vi "判决.vi"(1 "判决门限":dbl, 2 "噪声数组":dbl[](array[numeric]), 3 "码元数组":dbl[](array[numeric])) -> (0 "错误计数":dbl)   [LabVIEW 2020]
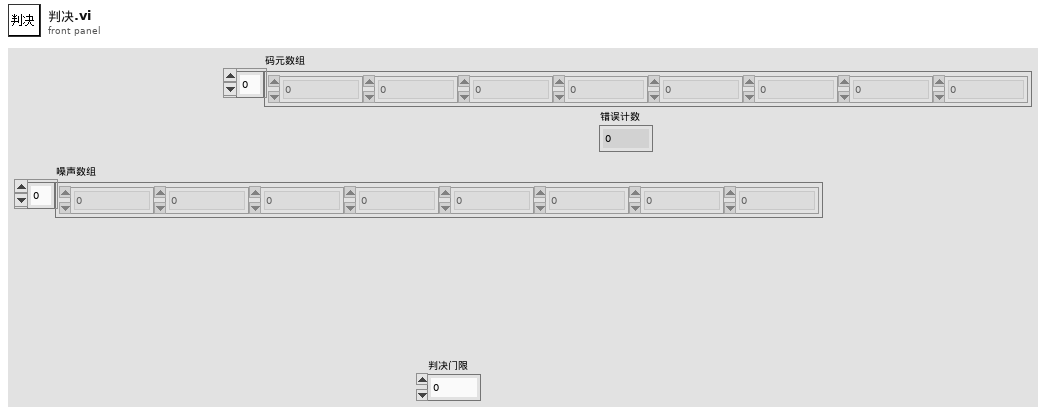
[diagram p1: front panel]
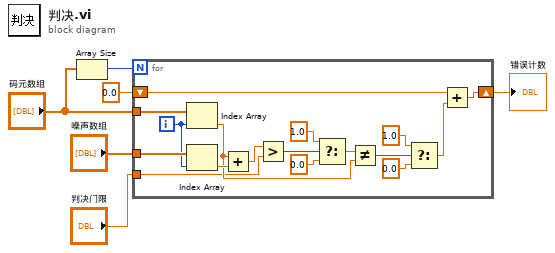
[diagram p0: block diagram]
diagram:
  n1 = Array Size(array="码元数组") -> (size(s)=w1:i32)
  n2 = for {
    N: w1 -> [_]
    tunnel: "噪声数组" -> [w19]
    shift-right: [w13] -> w3
    shift-left: 0.0 -> [w14]
    tunnel: "码元数组" -> [w8]
    tunnel: "判决门限" -> [w7]
    i -> [w10]
    n3 = Index Array(array=w8, index=w10) -> (element=w9:dbl)
    n4 = Index Array(array=w19, index=w10) -> (element=w11:dbl)
    n5 = Add(x=w9, y=w11) -> (x+y=w12:dbl)
    n6 = Greater?(x=w12, y=w7) -> (0:w21:bool)
    n7 = Select(t=1.0, s=w21, f=0.0) -> (s? t:f=w20:dbl)
    n8 = Not Equal?(x=w20, y=w9) -> (x != y?=w18:bool)
    n9 = Select(t=1.0, s=w18, f=0.0) -> (s? t:f=w15:dbl)
    n10 = Add(x=w14, y=w15) -> (x+y=w13:dbl)
  }
  "错误计数" <- w3
